vi "Optim joy manipulator.vi"(11 "device index":i32=7) -> (0 "error out":errorcluster, 1 "POV":bool, 3 "Refnum out":refnum<k1>, 4 "Cluster":T4, 5 "wysylanie":bool, 7 "axis info":T3)   [LabVIEW 2014]
uses:
  <vilib>/Utility/inputDevices.llb/joystickAcquire.vi
panel:
  out "direction info":T1
  out "button info":T2
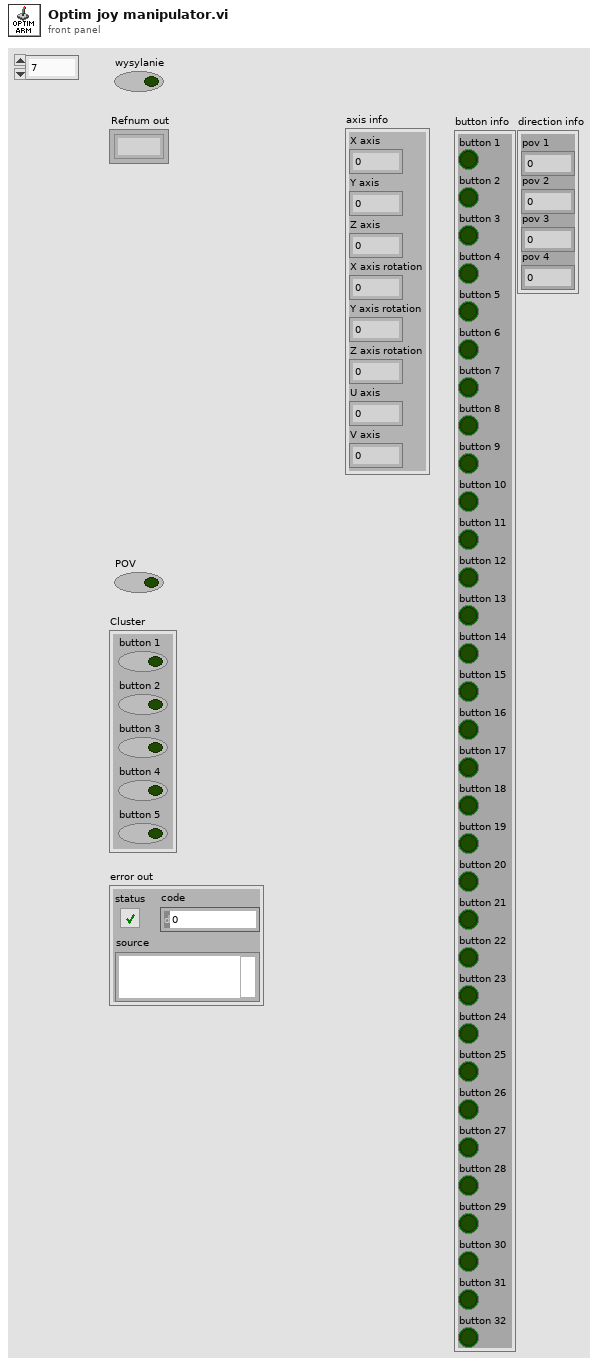
[diagram p1: front panel]
types:
  T1 = cluster{"pov 1":i32, "pov 2":i32, "pov 3":i32, "pov 4":i32}
  T2 = cluster{"button 1":bool, "button 2":bool, "button 3":bool, "button 4":bool, "button 5":bool, "button 6":bool, "button 7":bool, "button 8":bool, "button 9":bool, "button 10":bool, "button 11":bool, "button 12":bool, "button 13":bool, "button 14":bool, "button 15":bool, "button 16":bool, "button 17":bool, "button 18":bool, "button 19":bool, "button 20":bool, "button 21":bool, "button 22":bool, "button 23":bool, "button 24":bool, "button 25":bool, "button 26":bool, "button 27":bool, "button 28":bool, "button 29":bool, "button 30":bool, "button 31":bool, "button 32":bool}
  T3 = cluster{"X axis":i32, "Y axis":i32, "Z axis":i32, "X axis rotation":i32, "Y axis rotation":i32, "Z axis rotation":i32, "U axis":i32, "V axis":i32}
  T4 = cluster{"button 1":bool, "button 2":bool, "button 3":bool, "button 4":bool, "button 5":bool}
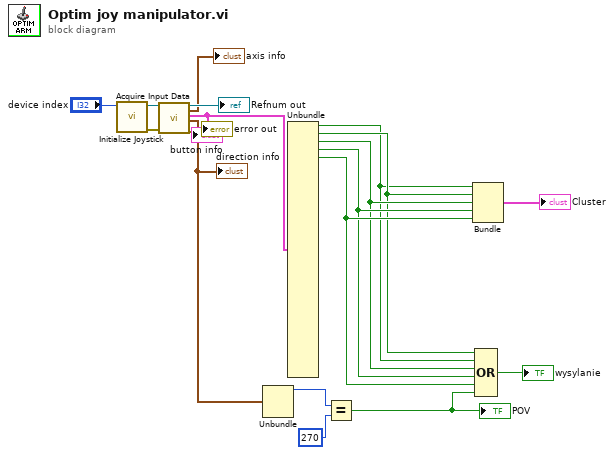
[diagram p0: block diagram]
diagram:
  n1 = call <vilib>:"Initialize Joystick.vi"("device index"="device index") -> ("error out"=w9:errorcluster, "device ID"=w1:refnum<k1>)  [unwired: 9 in]
  n2 = call-poly <vilib>:"Acquire Input Data.vi"("device ID"=w1, "error in (no error)"=w9) -> ("device ID"=→"Refnum out":refnum<k1>, "axis info"=→"axis info":T3, "button info"=w3:T2, "direction info"=w10:T1, "error out"=→"error out":errorcluster)  [unwired: 13 in]
  "button info" <- w3
  "direction info" <- w10
  n3 = Unbundle(w10) -> ("pov 1"=w4:i32)  [unwired: 3 out]
  n4 = Unbundle(w3) -> ("button 1"=w13:bool, "button 2"=w14:bool, "button 3"=w15:bool, "button 4"=w16:bool, "button 5"=w17:bool)  [unwired: 27 out]
  n5 = Equal?(x=w4, y=270) -> (x = y?=w12:bool)
  "POV" <- w12
  n6 = Bundle("button 1"=w13, "button 2"=w14, "button 3"=w15, "button 4"=w16, "button 5"=w17) -> (→"Cluster":T4)  [unwired: 1 in]
  n7 = Compound Arithmetic op=OR(w14, w13, w15, w16, w17, w12) -> (→"wysylanie":bool)
